vi "Get Alignment by Type.vi"(8 "error in (no error)":errorcluster, 11 "type":T1=enum."Void") -> (0 "error out":errorcluster, 3 "byte_alignment":i16)   [LabVIEW 2021, in "DataTypes_CIF_U.lvlib"]
uses:
  DataTypes_CIF_U.lvlib
  <vilib>/Utility/Data Type/Type Definitions/Data Type.ctl
  46e771c0-7912-4ce6-b3e3-2390ff6a635b.vi
  aacf5886-4db7-462f-891e-615d3d12e981.vi
  14245ff3-3107-41a2-8415-0aaa3f23f050.vi
  e78fac98-dca1-41d1-9ab5-e958f333f6f7.vi
  f593dffe-76a5-45ff-b122-289d97e0f02a.vi
  c27d18bf-49b0-434d-b50c-0bc95a9b75e4.vi
  997c4620-b9d7-4d59-bf2a-b666512fd16e.vi
  58474189-54be-4c19-acfd-aa5583055f53.vi
  3cfc3e04-3526-4e6a-aa5f-5a6b59df192c.vi
  e1be7635-64d7-4393-927b-34ed79dbbafe.vi
  74ca8250-03ce-42af-81e7-95331bf1f6cc.vi
  d55e1cdb-2dee-432b-914a-f3aa46316d74.vi
  8dc6945a-6818-43a5-bd3e-db50d7db5b0f.vi
  3379e68c-10ed-4b29-97f2-8f5e690714ae.vi
  a549c1ed-f632-448e-b564-78350d1b5bb2.vi
  e48eb750-bd78-443c-8be7-cd2515a4844b.vi
  3ee3f7aa-e930-4717-9752-ab1f2969e2ca.vi
  46e771c0-7912-4ce6-b3e3-2390ff6a635b.vi/7a63caab-3905-4750-8bef-3ed6d8464949.vi
  46e771c0-7912-4ce6-b3e3-2390ff6a635b.vi/ffc2c926-dd68-4b2a-8345-bf3c85a36d62.vi
  aacf5886-4db7-462f-891e-615d3d12e981.vi/7a63caab-3905-4750-8bef-3ed6d8464949.vi
  aacf5886-4db7-462f-891e-615d3d12e981.vi/ffc2c926-dd68-4b2a-8345-bf3c85a36d62.vi
  14245ff3-3107-41a2-8415-0aaa3f23f050.vi/7a63caab-3905-4750-8bef-3ed6d8464949.vi
  14245ff3-3107-41a2-8415-0aaa3f23f050.vi/ffc2c926-dd68-4b2a-8345-bf3c85a36d62.vi
  e78fac98-dca1-41d1-9ab5-e958f333f6f7.vi/7a63caab-3905-4750-8bef-3ed6d8464949.vi
  e78fac98-dca1-41d1-9ab5-e958f333f6f7.vi/ffc2c926-dd68-4b2a-8345-bf3c85a36d62.vi
  f593dffe-76a5-45ff-b122-289d97e0f02a.vi/7a63caab-3905-4750-8bef-3ed6d8464949.vi
  f593dffe-76a5-45ff-b122-289d97e0f02a.vi/ffc2c926-dd68-4b2a-8345-bf3c85a36d62.vi
  c27d18bf-49b0-434d-b50c-0bc95a9b75e4.vi/7a63caab-3905-4750-8bef-3ed6d8464949.vi
  c27d18bf-49b0-434d-b50c-0bc95a9b75e4.vi/ffc2c926-dd68-4b2a-8345-bf3c85a36d62.vi
  997c4620-b9d7-4d59-bf2a-b666512fd16e.vi/7a63caab-3905-4750-8bef-3ed6d8464949.vi
  997c4620-b9d7-4d59-bf2a-b666512fd16e.vi/ffc2c926-dd68-4b2a-8345-bf3c85a36d62.vi
  58474189-54be-4c19-acfd-aa5583055f53.vi/7a63caab-3905-4750-8bef-3ed6d8464949.vi
  58474189-54be-4c19-acfd-aa5583055f53.vi/ffc2c926-dd68-4b2a-8345-bf3c85a36d62.vi
  3cfc3e04-3526-4e6a-aa5f-5a6b59df192c.vi/7a63caab-3905-4750-8bef-3ed6d8464949.vi
  3cfc3e04-3526-4e6a-aa5f-5a6b59df192c.vi/ffc2c926-dd68-4b2a-8345-bf3c85a36d62.vi
  e1be7635-64d7-4393-927b-34ed79dbbafe.vi/7a63caab-3905-4750-8bef-3ed6d8464949.vi
  e1be7635-64d7-4393-927b-34ed79dbbafe.vi/ffc2c926-dd68-4b2a-8345-bf3c85a36d62.vi
  74ca8250-03ce-42af-81e7-95331bf1f6cc.vi/7a63caab-3905-4750-8bef-3ed6d8464949.vi
  74ca8250-03ce-42af-81e7-95331bf1f6cc.vi/ffc2c926-dd68-4b2a-8345-bf3c85a36d62.vi
  d55e1cdb-2dee-432b-914a-f3aa46316d74.vi/7a63caab-3905-4750-8bef-3ed6d8464949.vi
  d55e1cdb-2dee-432b-914a-f3aa46316d74.vi/ffc2c926-dd68-4b2a-8345-bf3c85a36d62.vi
  8dc6945a-6818-43a5-bd3e-db50d7db5b0f.vi/7a63caab-3905-4750-8bef-3ed6d8464949.vi
  8dc6945a-6818-43a5-bd3e-db50d7db5b0f.vi/ffc2c926-dd68-4b2a-8345-bf3c85a36d62.vi
  3379e68c-10ed-4b29-97f2-8f5e690714ae.vi/7a63caab-3905-4750-8bef-3ed6d8464949.vi
  3379e68c-10ed-4b29-97f2-8f5e690714ae.vi/ffc2c926-dd68-4b2a-8345-bf3c85a36d62.vi
  a549c1ed-f632-448e-b564-78350d1b5bb2.vi/7a63caab-3905-4750-8bef-3ed6d8464949.vi
  a549c1ed-f632-448e-b564-78350d1b5bb2.vi/ffc2c926-dd68-4b2a-8345-bf3c85a36d62.vi
  e48eb750-bd78-443c-8be7-cd2515a4844b.vi/7a63caab-3905-4750-8bef-3ed6d8464949.vi
  e48eb750-bd78-443c-8be7-cd2515a4844b.vi/ffc2c926-dd68-4b2a-8345-bf3c85a36d62.vi
  3ee3f7aa-e930-4717-9752-ab1f2969e2ca.vi/7a63caab-3905-4750-8bef-3ed6d8464949.vi
  3ee3f7aa-e930-4717-9752-ab1f2969e2ca.vi/ffc2c926-dd68-4b2a-8345-bf3c85a36d62.vi
  Typedef/Errors.ctl
  <vilib>/Utility/Data Type/NI_Data Type.lvlib
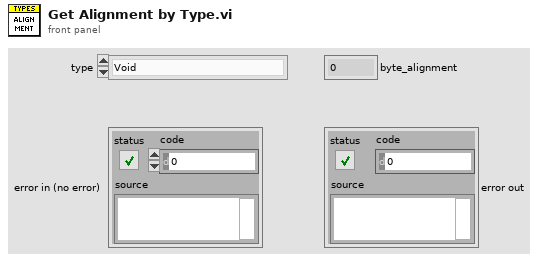
[diagram p1: front panel]
types:
  T1 = typedef "NI_Data Type.lvlib/Data Type.ctl" = enum8{"Invalid Type", "Void", "I8", "I16", "I32", "I64", "U8", "U16", "U32", "U64", "Single Float", "Double Float", "Extended Float", "Single Complex", "Double Complex", "Extended Complex", "Enum U8", "Enum U16", "Enum U32", "Enum U64", "Single Float With Unit", "Double Float With Unit", "Extended Float With Unit", "Single Complex with Unit", "Double Complex with Unit", "Extended Complex with Unit", "Boolean", "String", "Path", "Picture", "Tag", "Array", "Cluster", "Variant", "LV Variant", "Waveform", "Timestamp", "Digital Waveform", "Digital Data", "ExpressData", "Refnum", "External Data", "VI", "Poly VI", "LabVIEW Class Instance", "Fixed Point", "Set Collection", "Map Collection"}
  T2 = typedef "DataTypes_CIF_U.lvlib/Errors.ctl" = enum16{"Too few bytes", "Unsupported Type"}
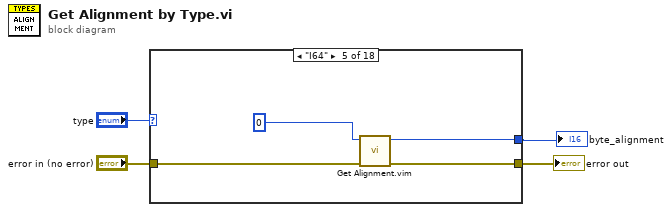
[diagram p0: block diagram]
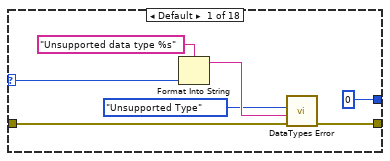
[diagram p2: hidden frame]
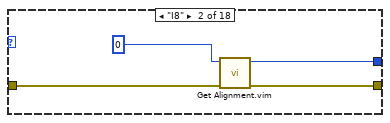
[diagram p3: hidden frame]
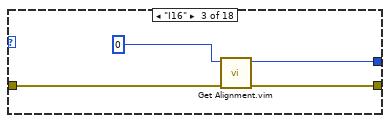
[diagram p4: hidden frame]
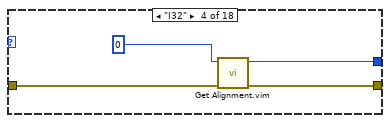
[diagram p5: hidden frame]
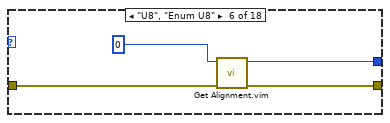
[diagram p6: hidden frame]
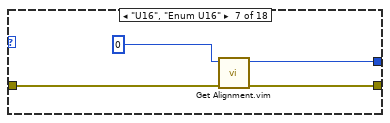
[diagram p7: hidden frame]
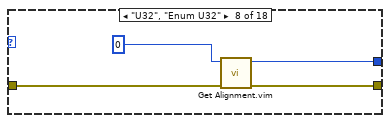
[diagram p8: hidden frame]
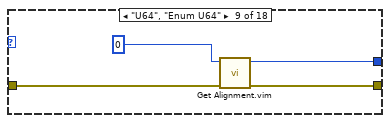
[diagram p9: hidden frame]
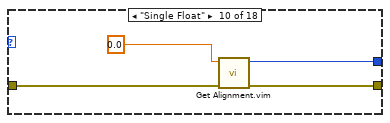
[diagram p10: hidden frame]
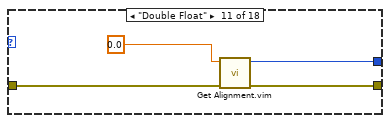
[diagram p11: hidden frame]
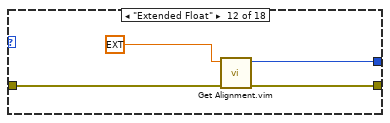
[diagram p12: hidden frame]
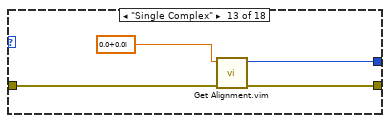
[diagram p13: hidden frame]
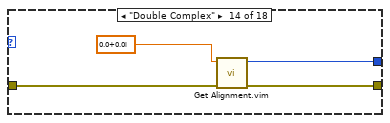
[diagram p14: hidden frame]
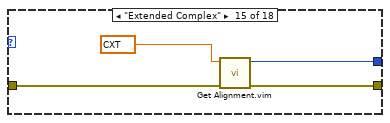
[diagram p15: hidden frame]
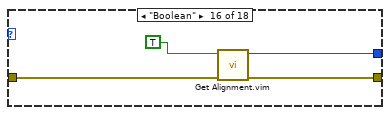
[diagram p16: hidden frame]
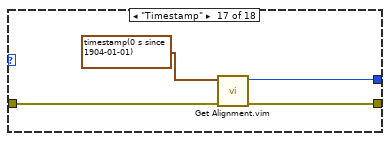
[diagram p17: hidden frame]
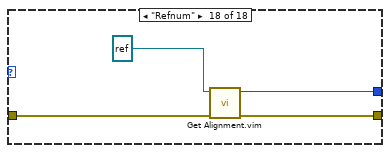
[diagram p18: hidden frame]
diagram:
  n1 = case shown="\"I64\"" "type" {
    selector: "type" -> [w6 _ _ _ _ _ _ _ _ _ _ _ _ _ _ _ _ _]
    tunnel: "error in (no error)" -> [w5 w15 w19 w23 w25 w29 w32 w37 w40 w44 w48 w52 w56 w60 w65 w70 w73 w79]
    tunnel: [w7 w14 w16 w20 w24 w28 w33 w36 w41 w45 w49 w53 w57 w61 w64 w69 w72 w77] -> w3
    tunnel: [i16 0 ("mem_size") w12 w17 w21 w26 w30 w34 w38 w42 w46 w50 w54 w58 w62 w66 w68 w74 w76] -> w1
    frame Default {
      n2 = Format Into String(format string="Unsupported data type %s", w6) -> (resulting string=w10:string)  [unwired: 2 in, 1 out]
      n3 = call "DataTypes Error.vi"("error in (no error)"=w5, "String to Append"=w10, "Error"=Errors."Unsupported Type") -> ("error out"=w7:errorcluster)  [unwired: 8 in]
    }
    frame "I8" {
      n4 = call "Get Alignment.vim"("error in (no error)"=w15, "data"=i8 0) -> ("error out"=w14:errorcluster, "byte_alignment"=w12:i16)  [unwired: 8 in]
    }
    frame "I16" {
      n5 = call "Get Alignment.vim"("error in (no error)"=w19, "data"=i16 0) -> ("error out"=w16:errorcluster, "byte_alignment"=w17:i16)  [unwired: 8 in]
    }
    frame "I32" {
      n6 = call "Get Alignment.vim"("error in (no error)"=w23, "data"=0) -> ("error out"=w20:errorcluster, "byte_alignment"=w21:i16)  [unwired: 8 in]
    }
    frame "I64" {
      n7 = call "Get Alignment.vim"("error in (no error)"=w25, "data"=i64 0) -> ("error out"=w24:errorcluster, "byte_alignment"=w26:i16)  [unwired: 8 in]
    }
    frame "U8", "Enum U8" {
      n8 = call "Get Alignment.vim"("error in (no error)"=w29, "data"=u8 0) -> ("error out"=w28:errorcluster, "byte_alignment"=w30:i16)  [unwired: 8 in]
    }
    frame "U16", "Enum U16" {
      n9 = call "Get Alignment.vim"("error in (no error)"=w32, "data"=u16 0) -> ("error out"=w33:errorcluster, "byte_alignment"=w34:i16)  [unwired: 8 in]
    }
    frame "U32", "Enum U32" {
      n10 = call "Get Alignment.vim"("error in (no error)"=w37, "data"=u32 0) -> ("error out"=w36:errorcluster, "byte_alignment"=w38:i16)  [unwired: 8 in]
    }
    frame "U64", "Enum U64" {
      n11 = call "Get Alignment.vim"("error in (no error)"=w40, "data"=u64 0) -> ("error out"=w41:errorcluster, "byte_alignment"=w42:i16)  [unwired: 8 in]
    }
    frame "Single Float" {
      n12 = call "Get Alignment.vim"("error in (no error)"=w44, "data"=sgl 0.0) -> ("error out"=w45:errorcluster, "byte_alignment"=w46:i16)  [unwired: 8 in]
    }
    frame "Double Float" {
      n13 = call "Get Alignment.vim"("error in (no error)"=w48, "data"=0.0) -> ("error out"=w49:errorcluster, "byte_alignment"=w50:i16)  [unwired: 8 in]
    }
    frame "Extended Float" {
      n14 = call "Get Alignment.vim"("error in (no error)"=w52, "data"=ext 0.0) -> ("error out"=w53:errorcluster, "byte_alignment"=w54:i16)  [unwired: 8 in]
    }
    frame "Single Complex" {
      n15 = call "Get Alignment.vim"("error in (no error)"=w56, "data"=csg 0.0+0.0i) -> ("error out"=w57:errorcluster, "byte_alignment"=w58:i16)  [unwired: 8 in]
    }
    frame "Double Complex" {
      n16 = call "Get Alignment.vim"("error in (no error)"=w60, "data"=cdb 0.0+0.0i) -> ("error out"=w61:errorcluster, "byte_alignment"=w62:i16)  [unwired: 8 in]
    }
    frame "Extended Complex" {
      n17 = call "Get Alignment.vim"("error in (no error)"=w65, "data"=cxt 0.0+0.0i) -> ("error out"=w64:errorcluster, "byte_alignment"=w66:i16)  [unwired: 8 in]
    }
    frame "Boolean" {
      n18 = call "Get Alignment.vim"("error in (no error)"=w70, "data"=TRUE) -> ("error out"=w69:errorcluster, "byte_alignment"=w68:i16)  [unwired: 8 in]
    }
    frame "Timestamp" {
      n19 = call "Get Alignment.vim"("error in (no error)"=w73, "data"=timestamp(0 s since 1904-01-01) ("Time Stamp")) -> ("error out"=w72:errorcluster, "byte_alignment"=w74:i16)  [unwired: 8 in]
    }
    frame "Refnum" {
      n20 = call "Get Alignment.vim"("error in (no error)"=w79, "data"=refnum<file> refnum) -> ("error out"=w77:errorcluster, "byte_alignment"=w76:i16)  [unwired: 8 in]
    }
  }
  "error out" <- w3
  "byte_alignment" <- w1
